vi "Generate control system simulated cycle.vi"(9 "ROI Dwell time (us)":dbl=4.0 min=0.05 max=20.0 step=0.05, 10 "Control system time resolution (0.05us)":dbl=0.05, 11 "Number of POI":i32=3) -> (3 "Simulated control timings sequence":waveform(dbl)(graph))   [LabVIEW 2013]
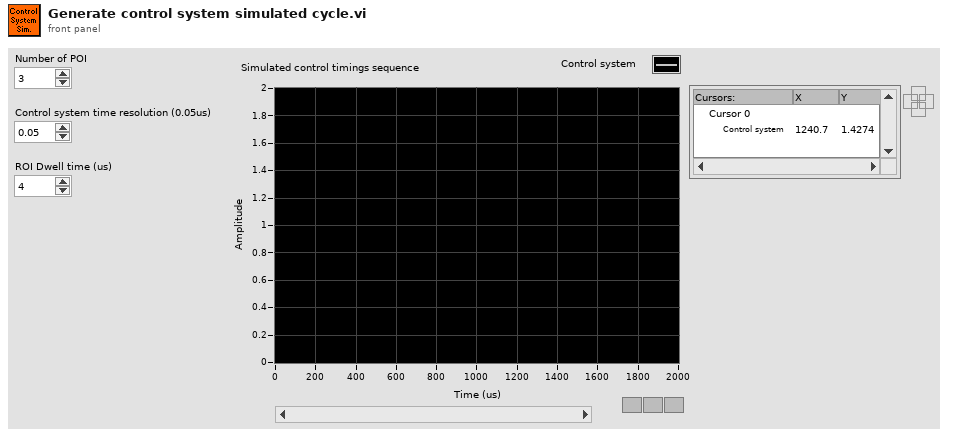
[diagram p1: front panel]
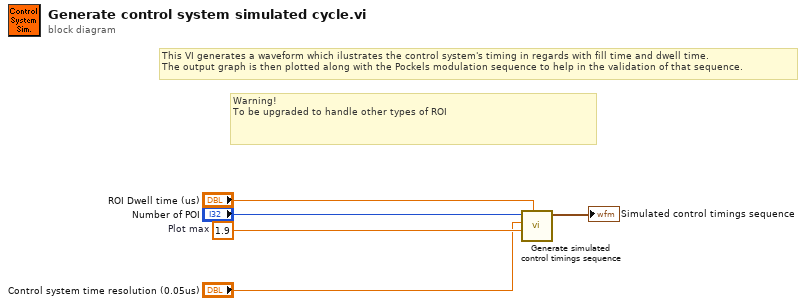
[diagram p0: block diagram]
diagram:
  w3 = 1.9  # Plot max
  # "This VI generates a waveform which ilustrates the control system's timing in regards with fill time and dwell time.\nThe output graph is then plotted along with the Pockels modulation sequence to help in the validation of that sequence."
  # "Warning!\nTo be upgraded to handle other types of ROI"
  n1 = call "Generate simulated control timings sequence.vi"("ROI Dwell time"="ROI Dwell time (us)", "High value of simulated waveform"=w3, "Time resolution of simulated waveform"="Control system time resolution (0.05us)", "Number of POI"="Number of POI") -> ("Simulated control timings sequence in"=→"Simulated control timings sequence":waveform(dbl))  [unwired: 7 in]
